vi "Get ID.vi"(11 "Interface in":refnum<class "Interface.lvclass">) -> (2 "ID":i32, 3 "Interface out":refnum<class "Interface.lvclass">)   [LabVIEW 2019, in "DSF Core.lvlib" / "Interface.lvclass"]
uses:
  Interface.lvclass
  Interface.lvclass/Interface.ctl
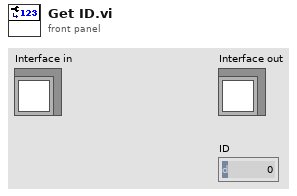
[diagram p1: front panel]
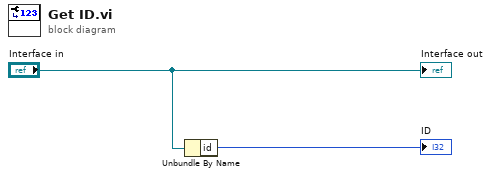
[diagram p0: block diagram]
diagram:
  n1 = Unbundle By Name("Interface in") -> ("id"=→"ID":i32)
  "Interface out" <- "Interface in"
